vi "HFRR ADV v09.vi"() -> ()   [LabVIEW 2025] (continued)
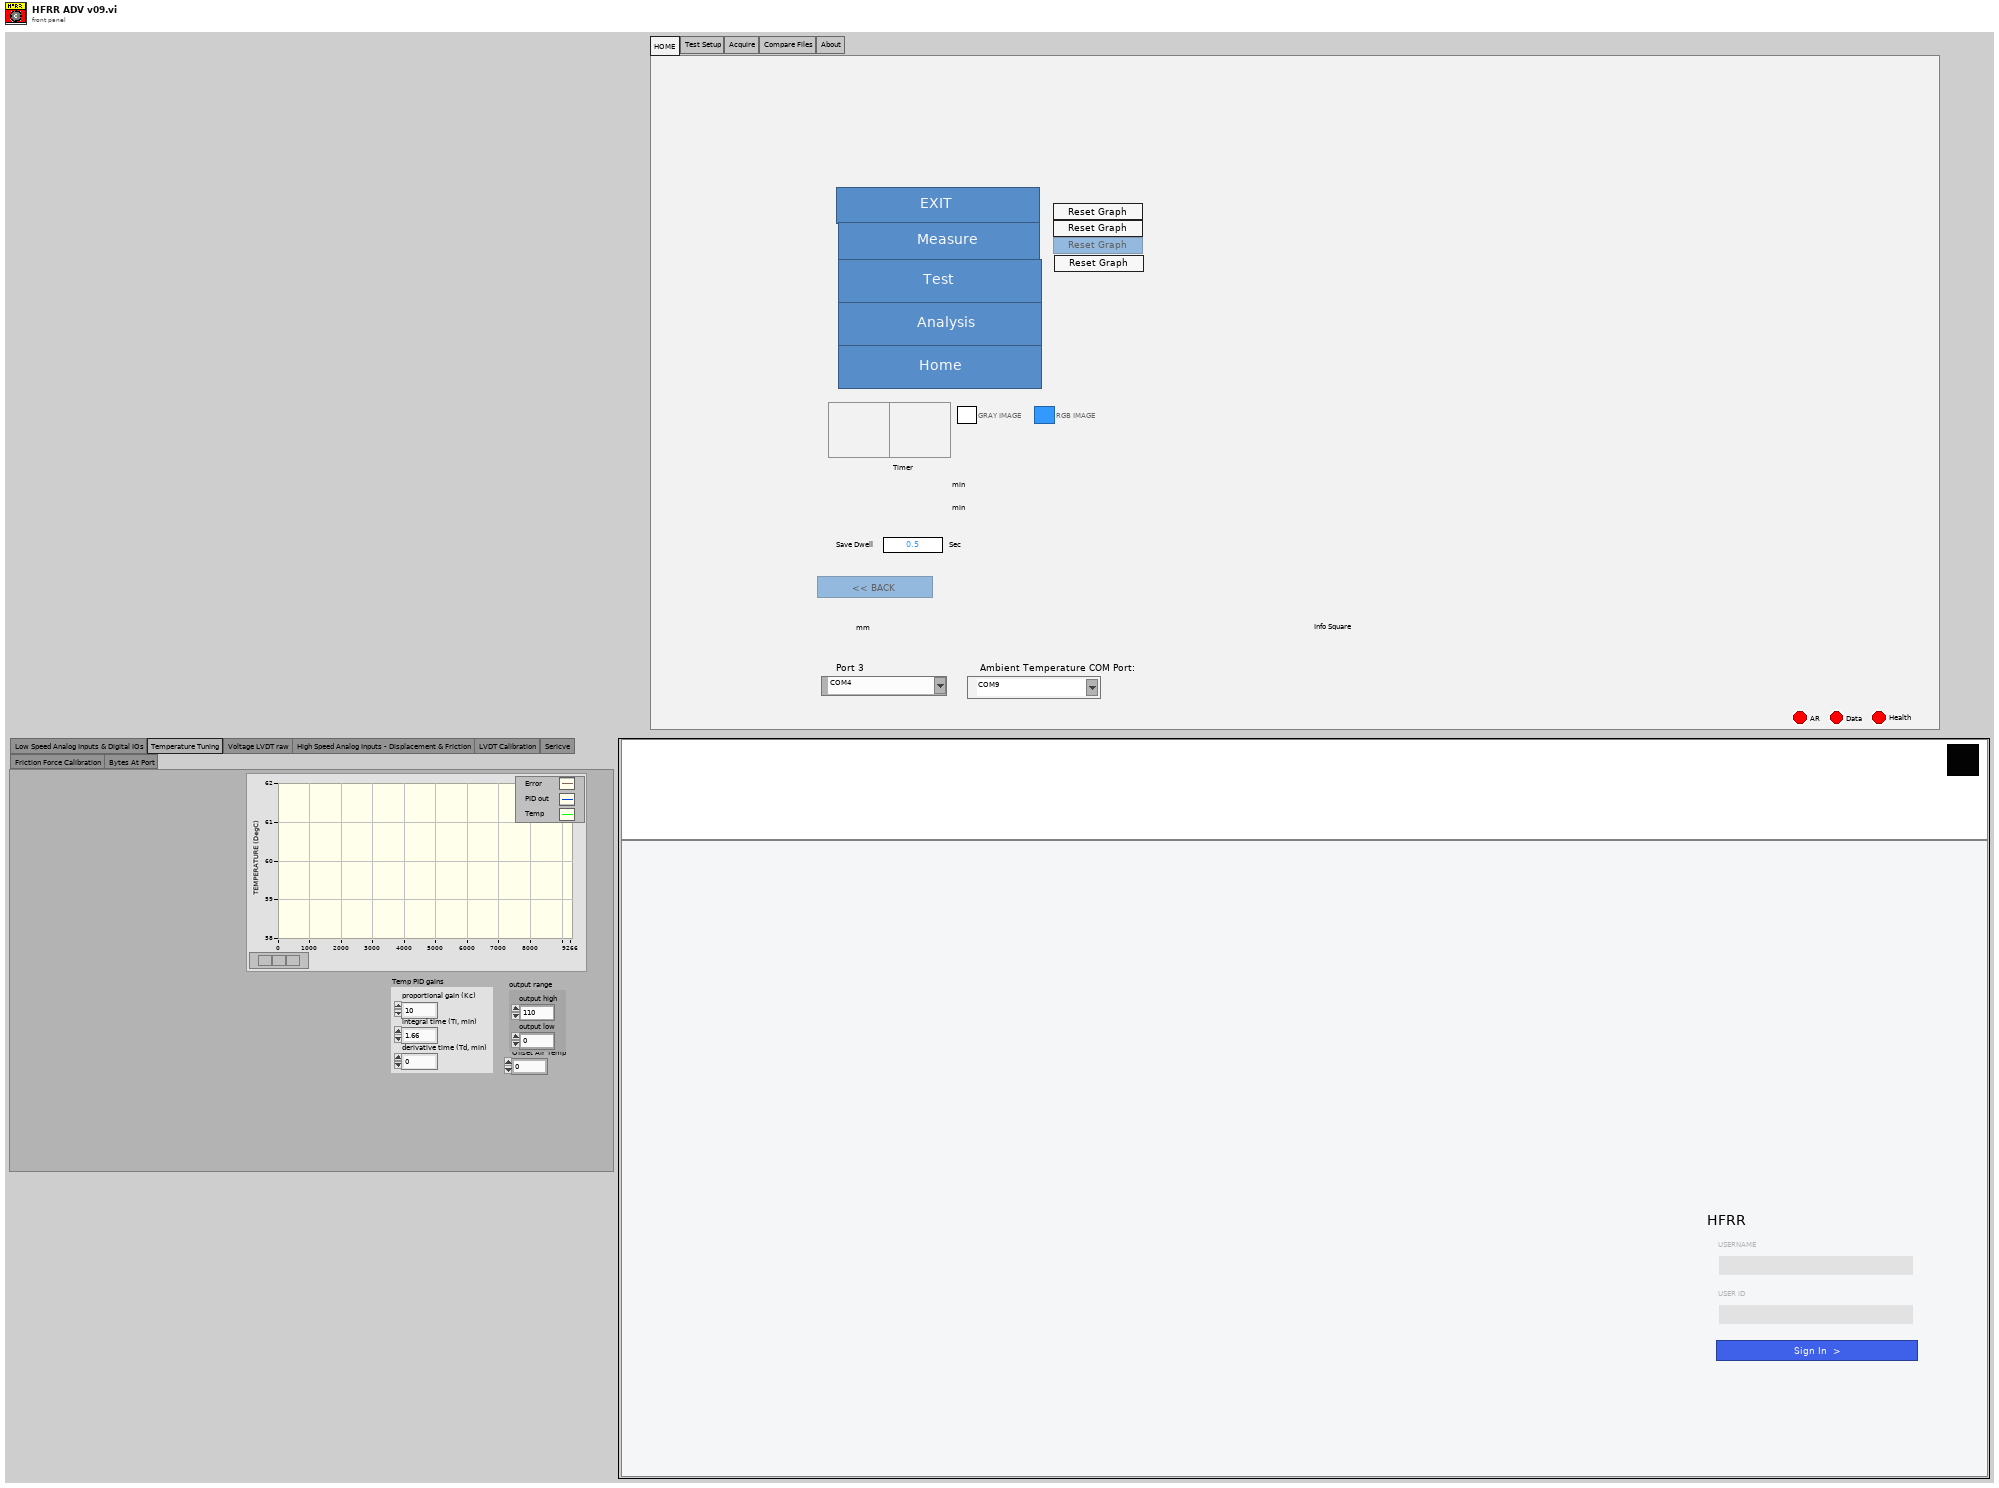
[diagram p1: front panel]
types:
  T1 = enum32{"Home", "Dashboard", "Imaging", "Report", "Analysis", "About", "Test Setup", "Advance"}
  T2 = enum32{"HOME", "Test Setup", "Acquire", "Adv Scar", "Adv Scar Report", "Compare Files", "About", "Advance", "Mooha"}
  T3 = enum16{"ASTM D6079", "ISO 12156", "CEC F-096-A-06", "Custom"}
  T4 = enum32{"Dashboard 1", "Dashboard 2", "Dashboard 3"}
  T5 = enum32{"COF", "Friction", "ECR", "Temperature", "Humidity", "Stroke"}
  T6 = enum32{"Coefficient Of Friction", "Air Temperature", "Humidity", "Stroke", "Sample Temperature", "Electrical Contact Resistance", "Frequency", "Air Temp vs Rh"}
  T7 = enum32{"Stroke Data", "Temperature Calibration", "Friction Force Raw Data"}
  T8 = cluster{"Proportional Gain (Kc)":dbl, "Integral Time (Ti, min)":dbl, "Derivative Time (Td, min)":dbl}
  T9 = enum32{"Temp Variables", "Camera", "WO 2465 (1)", "WO 2465 (2)", "WO 2465 (3)"}
  T10 = typedef "Auto Start enum.ctl" = enum16{"Init", "Humidity & Temperature On", "Reach point", "Maintain Stage", "Start Stage", "close", "Exit"}
  T11 = enum32{"Freqz control", "Low Speed Analog Inputs & Digital IOs", "Temperature Tuning", "Voltage LVDT raw", "High Speed Analog Inputs - Displacement & Friction", "LVDT Calibration", "Sericve", "Friction Force Calibration", "Bytes At Port", "Loadcell Board"}
  T12 = cluster{"proportional gain (Kc)":dbl, "integral time (Ti, min)":dbl, "derivative time (Td, min)":dbl}
  T13 = typedef "imagedata.ctl" = cluster{"image type":i32, "image depth":i32, "image":u8[], "mask":u8[], "colors":u32[], "Rectangle":cluster{"left":i16, "top":i16, "right":i16, "bottom":i16}}
  T14 = enum32{"HOME", "Test Setup", "Acquire", "Compare Files", "Print Report", "About", "Advance", "Mooha"}
  T15 = enum8{"Enabled", "Disabled", "Disabled and Grayed Out"}
  T16 = cluster{"Read Heave and Surge":string, "Bytes at Heave Port":dbl, "Heave and Surge COM Port:":refnum<visa-resource-name>, "Com Port 2":refnum<visa-resource-name>, "Residual Due":string, "Heave COM Status 2":bool, "Heave COM Status":bool, "Port 2":bool, "Sway PPR":dbl, "Surge PPR":dbl, "Heave PPR":dbl, "Sway Pitch":dbl, "Surge Pitch":dbl, "Heave Pitch":dbl, "Sway Pulses/mm":dbl, "Surge Pulses/mm":dbl, "Heave Pulses/mm":dbl, "inner loop":dbl, "Read Heave and Surge 2":string, "String 36":string, "Write S":bool, "WriteCC1":string[], "Heave COM Loop":i32, "LastCom":string, "EXIT":bool, "Error Heave":errorcluster}
  T17 = enum16{"Always On", "Always Off", "Off While Running"}
  T18 = typedef "POST ANALYSIS ENUM.ctl" = enum16{"OPEN EXE", "INIT", "OPEN FILE", "FIT", "DRAW REC", "DRAW LINE", "PAN", "ZOOM IN", "ZOOM OUT", "SET ZOOM", "CLEAR ROI", "GET MEASUREMENTS", "RESIZE MODE", "STREAM START", "STREAM STOP", "SHOW UI", "MINIMIZE UI", "HIDE UI", "CKISE APP", "CLOSE CONNECTION", "SAVE IMAGE", "SET ROI COLOR", "READ", "TCP CHECK", "CLOSE"}
  T19 = typedef "CAMERA LIVE FEED ENUM.ctl" = enum16{"OPEN EXE", "INIT", "READ", "CAMERA CONNECT", "CAMERA START", "CAMERA STOP", "CAMERA GRAY", "CAMERA RGB", "CAMERA MINIMIZE", "CAMERA CLOSE", "CAMERA MODE LIST", "CAMERA MODE SET", "CAMERA RESTORE", "CAMERA SAVE", "CLOSE"}
  T20 = cluster{"File Name":string, "Test Method":string, "Operator":string, "Fuel Description":string, "Date and time":string}
  T21 = enum32{"Home", "Dashboard", "Imaging", "Report", "Analysis", "About", "Test Setup"}
  T22 = enum32{"HOME", "Test Setup", "Acquire", "Compare Files", "About", "Advance", "Mooha"}
  T23 = enum16{"deny read/write", "deny write-only", "deny none"}
  T24 = typedef "NI_ReportGenerationCore.lvlib/HTML Report Image Alignment.ctl" = enum16{"(default)", "LEFT", "RIGHT", "TOP", "TEXTTOP", "MIDDLE", "ABSMIDDLE", "BASELINE", "BOTTOM", "ABSBOTTOM"}
  T25 = enum16{"open", "replace", "create", "open or create", "replace or create", "replace or create with confirmation"}
  T26 = enum16{"INIT", "READ", "MANUAL WRITE", "WRITE", "CLOSE", "ERROR INIT"}
  T27 = enum16{"open", "open or create", "create or replace", "create", "open (read only)"}
  T28 = cluster{"Mode":enum16{"RTU", "ASCII"}, "Slave Address":u8}
diagram:
  w1 = T15."Enabled" ("Disabled")
  w4 = FALSE ("Visible")
  w3 = FALSE ("Humidity Off Command")
  w23 = "" ("USER ID")
  # "[CH1]    - FF\n[CH2]   - TEMPERATURE\n[CH3]    - Humidity\n[CH4]    - AIR TEMP\n[CH5]\\- Visa Uno\n[CH6] \\- Visa Due\n[CH7]  \\- file path\n[CH8]   - Displacement Gain\n[CHA]   - Stroke Gain\n[CHB]   - Stroke PID Gain\n[CHC]   -Language Selection\n[CHD]   -Power +\n[CHE]   -Power_\n[CHF]   -Heater\n[CHG]   -Humidity Wet\n[CHH]   -Humidity Dry\n[CHI]   -Integral Time \n[CHIJ   -Air intercept\n[CHI]   -Temp Intercept"
  n1 = flat-sequence {
    tunnel: [w78] -> w14
    tunnel: w14 -> [w92]
    tunnel: [w91] -> w13
    tunnel: ["ao0"] -> w16
    tunnel: w13 -> [_]
    tunnel: w16 -> [w157]
    tunnel: [w157] -> w15
    tunnel: w15 -> [w210]
    tunnel: [w208] -> w27
    tunnel: [w210] -> w26
    tunnel: w27 -> [w261]
    tunnel: w26 -> [w217]
    tunnel: [w261] -> w12
    tunnel: [w223] -> w11
    tunnel: [w211] -> w10
    tunnel: [w268] -> _
    tunnel: [w267] -> _
    tunnel: [w269] -> w55
    tunnel: w12 -> [w269]
    tunnel: w11 -> [w267]
    tunnel: w10 -> [w268]
    frame #0 {
      n2 = control-ref of="This VI"() -> (w66:refnum<vi>)
      n3 = property class="VI"(reference=w66) -> (reference out=w57:refnum<vi>, error out=w61:errorcluster, "Panel"=w65:refnum<vi>)  [unwired: 1 in]
      n4 = property class="Pnl"(reference=w65, error in=w61) -> (reference out=w59:refnum<vi>, error out=w62:errorcluster, "Panes[]"=w64:refnum<vi>[])
      n5 = for {
        tunnel: w64 -> [w72] mode=indexing
        tunnel: T17."Always Off" ("Horizontal Scrollbar Visibility") -> [w71]
        tunnel: w62 -> [w68]
        tunnel: [w67] -> w60
        n6 = property class="Pane"(reference=w72, error in=w68, "HorizScrollbarVisibility"=w71) -> (reference out=w69:refnum<vi>, error out=w70:errorcluster)
        n7 = Close Reference(reference=w69, error in (no error)=w70) -> (error out=w67:errorcluster)
      }
      n8 = Close Reference(reference=w59, error in (no error)=w60) -> (error out=w58:errorcluster)
      n9 = Close Reference(reference=w57, error in (no error)=w58) -> (error out=→"error out 8":errorcluster)
    }
    frame #1 {
      n10 = call "CLOSE CONNECTION.vi"("error in (no error)"="error in (no error) 2") -> ("error out"=w76:errorcluster)  [unwired: 10 in]
      n11 = call <vilib>:"Clear Errors.vi"("error in (no error)"=w76) -> ("error out"=w75:errorcluster)  [unwired: 5 in, 1 out]
      n12 = disable-structure shown="Enabled" {
        disable-tunnel: w75 -> [w82 _]
        disable-tunnel: [w81 _] -> w78
        frame Enabled {
          n13 = call <userlib>:"Fit VI window to Largest Dec.vi"("error in (no error)"=w82, "border spacing (2 px)"=1) -> ("error out"=w85:errorcluster, "dup VI Ref"=w89:refnum<vi>)  [unwired: 4 in]
          n14 = invoke on="Invoke Node" class="VI" method="FP.Run-Time Position.Maximized"(reference=w89, error in=w85) -> (error out=w86:errorcluster)  [unwired: 2 in, 3 out]
          n15 = call <vilib>:"Clear Errors.vi"("error in (no error)"=w86) -> ("error out"=w88:errorcluster)  [unwired: 5 in, 1 out]
          n16 = control-ref of="This VI"() -> (w80:refnum<vi>)
          n17 = invoke on="Invoke Node" class="VI" method="Default Vals.Reinit All"(reference=w80, error in=w88) -> (reference out=w84:refnum<vi>, error out=w83:errorcluster)  [unwired: 1 in, 1 out]
          n18 = Close Reference(reference=w84, error in (no error)=w83) -> (error out=w81:errorcluster)
        }
        frame Disabled {
        }
      }
      n19 = local write "sign in temp"(FALSE ("sign in temp")) -> ()
      n20 = property on="Sign In" class="Bool (strict)"("DisabledEnum"=T15."Disabled" ("Disabled")) -> ()  [unwired: 2 in, 2 out]
      n21 = property on="Auto Scar Check" class="Clust (strict)"("Visible"=TRUE) -> ()  [unwired: 2 in, 2 out]
    }
    frame #2 {
      n22 = call "dialog box.vi"("Status"="Before starting the test, verify that the microscope cable is connected.", "error in"=w92) -> ("error out"=w91:errorcluster)  [unwired: 8 in]
    }
    frame #3 {
      w99 = FALSE ("Upld AR 2")
      # "kkkkk"
      # "C:\\Windows\\wndcm_pw_stdED hfrr.txt"
      # "C:\\LAB-IQ NXT"
      # "C:\\LAB-IQ NXT\\wndcm_pw_stdED hfrr.txt"
      # "password file"
      n23 = Current VI's Path() -> (path=w112:path)
      n24 = Strip Path(path=w112) -> (stripped path=w105:path)  [unwired: 1 out]
      n25 = Path To String(path=w105) -> (string=w107:string)
      n26 = local write "conststatus"(0.0 ("rpm value : 2")) -> ()
      n27 = local write "Upld AR 2"(TRUE ("Upld AR 2")) -> ()
      n28 = local write "Lan flag"(0.0 ("Lan flag")) -> ()
      n29 = local write "COUNT"(0 ("COUNT")) -> ()
      n30 = local write "FLAG 2"(0.0 ("FLAG 2")) -> ()
      n31 = local write "Com flag"(u32 0 ("Com flag")) -> ()
      n32 = local write "Re-Initialise"(TRUE ("Re-Initialise")) -> ()
      n33 = local write "refresh flag"(FALSE ("refresh flag")) -> ()
      n34 = local write "Json St Flg"(w99) -> ()
      n35 = Search/Split String(string=w107, search string/char (-)=".exe") -> (match + rest of string=w109:string)  [unwired: 1 in, 2 out]
      n36 = Match True/False String(2:".vi" ("false string"), 3:".exe" ("true string"), 4:w109) -> (0:w106:bool)  [unwired: 1 out]
      n37 = local write "Json End Flg"(w99) -> ()
      n38 = case shown="True" w106 {
        tunnel: w105 -> [w128 w130]
        tunnel: [w128 w129] -> w103
        frame False {
        }
        frame True {
          n39 = Strip Path(path=w130) -> (stripped path=w129:path)  [unwired: 1 out]
        }
      }
      n40 = Path To String(path=w103) -> (string=→"Gain path":string)
      n41 = local write "Main Tab Display"(T4."Dashboard 1" ("Main Tab Display")) -> ()
      n42 = local write "main tab sub"(enum32{"Page 1", "Page 2"}."Page 1" ("main tab sub")) -> ()
      n43 = local write "Main Tab"(T2."HOME" ("Main Tab")) -> ()
      n44 = local write "EVENT LOG"("") -> ()
      n45 = List Folder(path=path "C:/LAB-IQ" ("directory path"), pattern="*.txt") -> (filenames=w118:string[])  [unwired: 2 in, 3 out]
      n46 = Search 1D Array(1D array=w118, element="wndcm_pw_stdED hfrr.txt") -> (index of element=w121:i32)  [unwired: 1 in]
      n47 = Equal?(x=w121, y=-1) -> (x = y?=w116:bool)
      n48 = case shown="True" w116 {
        frame False {
        }
        frame True {
          n49 = String To Byte Array(string="123\n") -> (unsigned byte array=w135:u8[])
          n50 = Array Size(array=w135) -> (size(s)=w134:i32)
          n51 = for {
            N: w134 -> [_]
            tunnel: w135 -> [w148]
            tunnel: [w145] -> w137 mode=indexing
            tunnel: w134 -> [w140]
            i -> [w138]
            n52 = Decrement(x=w140) -> (x-1=w141:i32)
            n53 = Equal?(x=w138, y=w141) -> (x = y?=w142:bool)
            n54 = Index Array(array=w148, index=w138) -> (element=w147:u8)
            n55 = Number To Decimal String(number=w147) -> (decimal integer string=w146:string)  [unwired: 1 in]
            n56 = Select(t="", s=w142, f="\r") -> (s? t:f=w139:string)
            n57 = Concatenate Strings(w146, w139) -> (w145:string)
          }
          n58 = local read "file path"() -> (w131:path)
          n59 = Concatenate Strings(w137) -> (w133:string)
          n60 = call <vilib>:"Write Characters To File.vi"("append to file? (new file:F)"=FALSE, "character string"=w133, "file path (dialog if empty)"=w131) -> ()  [unwired: 2 in, 1 out]
        }
      }
      n61 = local write "clk"(0.0 ("clk")) -> ()
      n62 = local write "Flag"(0.0 ("Flag")) -> ()
      "file path" <- path "C:/LAB-IQ/wndcm_pw_stdED hfrr.txt" ("file path")
      "FF buffer" <- dbl[] [] ("FF buffer")
    }
    frame #4 {
      # "C:\\WinDucom\\calibrate WO 2391.dcf"
      n63 = String To Path(string="C:\\LAB-IQ\\calibrate WO 2465.dcf") -> (path=w156:path)
      n64 = Open/Create/Replace File "Open File"(file path (use dialog)=w156) -> (refnum out=w155:refnum<file>)  [unwired: 5 in, 2 out]
      n65 = for {
        N: 24 -> [_]
        tunnel: w155 -> [w176]
        i -> [w170]
        (unwired) TRUE ("line mode (F)")
        n66 = Read from Text File "Read File"(file (use dialog)=w176) -> (text=w175:string)  [unwired: 3 in, 3 out]
        n67 = Match Pattern(string=w175, regular expression="]") -> (after substring=w173:string)  [unwired: 1 in, 3 out]
        n68 = String Subset(string=w175, offset (0)=5, length (rest)=10 ("length (rest)")) -> (substring=w168:string)
        n69 = Fract/Exp String To Number(string=w168) -> (number=w169:dbl)  [unwired: 3 in, 1 out]
        n70 = Match Pattern(string=w173, regular expression="-") -> (before substring=w171:string)  [unwired: 1 in, 3 out]
        n71 = case shown="7" w170 {
          tunnel: w169 -> [w179 w180 w181 w182 _ _ _ w187 w188 w189 w192 w193 w194 w195 w196 w197 w198 w201 w202 _ _ w205 _ _ _]
          tunnel: w171 -> [_ _ _ _ w183 w184 w185 _ _ _ _ _ _ _ _ _ _ _ _ w203 w204 _ w206 w207 _]
          frame 0 {
            n72 = local write "FRIC. FORCE :"(w179) -> ()
          }
          frame 1 {
            n73 = local write "TEMPERATURE :"(w180) -> ()
          }
          frame 2 {
            n74 = local write "HUMIDITY:"(w181) -> ()
          }
          frame 3 {
            n75 = local write "AIR TEMPERATURE :"(w182) -> ()
          }
          frame 4 {
            n76 = local write "Com Port 1"(w183) -> ()
          }
          frame 5 {
            n77 = local write "Com Port 2"(w184) -> ()
            n78 = local write "visa due"(w184) -> ()
          }
          frame 6 {
            n79 = String To Path(string=w185) -> (path=w186:path)
            n80 = local write "File Path"(w186) -> ()
          }
          frame 7 {
            n81 = local write "DISPLACEMENT :"(w187) -> ()
          }
          frame 8 {
            n82 = local write "STROKE GAIN :"(w188) -> ()
          }
          frame 9 {
            n83 = local read "Stroke PID Gains"() -> (w191:T8)
            n84 = Bundle By Name(cluster=w191, "Proportional Gain (Kc)"=w189) -> (w190:T8)
            n85 = local write "Stroke PID Gains"(w190) -> ()
          }
          frame 10 {
            n86 = local write "Language Selection"(w192) -> ()
          }
          frame 11 {
            n87 = local write "CH-POWER +"(w193) -> ()
          }
          frame 12 {
            n88 = local write "CH-POWER -"(w194) -> ()
          }
          frame 13 {
            n89 = local write "CH-HEATER"(w195) -> ()
          }
          frame 14 {
            n90 = local write "CH-HUMIDITY WET"(w196) -> ()
          }
          frame 15 {
            n91 = local write "CH-HUMIDITY DRY"(w197) -> ()
          }
          frame 16 {
            n92 = local read "Stroke PID Gains"() -> (w200:T8)
            n93 = Bundle By Name(cluster=w200, "Integral Time (Ti, min)"=w198) -> (w199:T8)
            n94 = local write "Stroke PID Gains"(w199) -> ()
          }
          frame 17 {
            n95 = local write "AIR TEMP INTERCEPT:"(w201) -> ()
          }
          frame 18 {
            n96 = local write "TEMP INTERCEPT:"(w202) -> ()
          }
          frame 19 {
            n97 = local write "S.NO"(w203) -> ()
          }
          frame 20 {
            n98 = local write "Com Port 3"(w204) -> ()
          }
          frame 21 {
            n99 = local write "LvdtOff"(w205) -> ()
          }
          frame 22 {
            n100 = local write "Humidity :"(w206) -> ()
          }
          frame 23 {
            n101 = local write "Camera Port :"(w207) -> ()
          }
          frame 24, Default {
          }
        }
      }
      n102 = String To Path(string="C:\\LAB-IQ\\Image Calibrate v01.dcf") -> (path=w152:path)
      n103 = Open/Create/Replace File ("Open File")(file path (use dialog)=w152) -> (refnum out=w151:refnum<file>)  [unwired: 5 in, 2 out]
      n104 = for {
        N: 4 -> [_]
        tunnel: w151 -> [w163]
        i -> [w159]
        n105 = Read from Text File ("Read File")(file (use dialog)=w163) -> (text=w164:string)  [unwired: 3 in, 3 out]
        n106 = String Subset(string=w164, offset (0)=6, length (rest)=10 ("length (rest)")) -> (substring=w160:string)
        n107 = Fract/Exp String To Number(string=w160) -> (number=w158:dbl)  [unwired: 3 in, 1 out]
        n108 = case shown="3" w159 {
          tunnel: w158 -> [w165 w166 _ w167 _]
          frame 0 {
            n109 = local write "5x Gain"(w165) -> ()
          }
          frame 1 {
            n110 = local write "10x Gain"(w166) -> ()
          }
          frame 2 {
          }
          frame 3 {
            n111 = local write "100x gain"(w167) -> ()
          }
          frame 4, Default {
          }
        }
      }
    }
    frame #5 {
      n112 = Wait (ms)(milliseconds to wait=u32 1000) -> (millisecond timer value=w208:u32)
    }
    frame #6 {
      w226 = u32 2000 ("milliseconds to wait")
      w253 = u32 2000 ("milliseconds to wait")
      n113 = local read "Re-Initialise"() -> (w260:bool)
      n114 = case shown="True" w260 {
        frame False {
        }
        frame True {
          n115 = local write "Re-Initialise"(FALSE ("Re-Initialise")) -> ()
        }
      }
      n116 = call "CAMERA LIVE FEED FGV.vi"("Enum - Menu"=CAMERA_LIVE_FEED_ENUM."OPEN EXE", "error in (no error)"=w217) -> ("error out"=w259:errorcluster)  [unwired: 8 in, 1 out]
      n117 = call "Stall Data Flow.vim"("value in"=w259, "milliseconds to wait"=w253) -> ("value out"=w257:errorcluster)  [unwired: 1 out]
      n118 = call "CAMERA LIVE FEED FGV.vi"("Enum - Menu"=CAMERA_LIVE_FEED_ENUM."INIT", "error in (no error)"=w257) -> ("error out"=w255:errorcluster)  [unwired: 8 in, 1 out]
      n119 = call "IMAGE ANALYSIS.vi"("Enum"=POST_ANALYSIS_ENUM."OPEN EXE", "error in"=w217) -> ("error out"=w214:errorcluster)  [unwired: 8 in, 1 out]
      n120 = case shown="Error .." w255 {
        selector: w255 -> [w262 _]
        tunnel: [w262 _] -> w254
        frame No Error {
        }
        frame Error {
          n121 = One Button Dialog(message="Camera initialization error.\nPlease Restart the software") -> ()  [unwired: 1 in, 1 out]
        }
      }
      n122 = call "Stall Data Flow.vim"("value in"=w214, "milliseconds to wait"=u32 8000) -> ("value out"=w213:errorcluster)  [unwired: 1 out]
      n123 = property on="Camera Port :" class="CmbBox"() -> ("Strings[]"=w251:string[], "Value"=w252:string)  [unwired: 2 in, 2 out]
      n124 = call "IMAGE ANALYSIS.vi"("Enum"=POST_ANALYSIS_ENUM."INIT", "error in"=w213) -> ("error out"=w211:errorcluster)  [unwired: 8 in, 1 out]
      n125 = Search 1D Array(1D array=w251, element=w252) -> (index of element=w250:i32)  [unwired: 1 in]
      n126 = Type Cast(type=30, x=w250) -> (*(type *) &x=w248:i32)
      n127 = call "Stall Data Flow.vim"("value in"=w254, "milliseconds to wait"=w253) -> ("value out"=w230:errorcluster)  [unwired: 1 out]
      n128 = Add(x=w248, y=48) -> (x+y=w229:i32)
      n129 = call "CAMERA LIVE FEED FGV.vi"("Enum - Menu"=CAMERA_LIVE_FEED_ENUM."CAMERA CONNECT", "error in (no error)"=w230, "CAMERA PORT"=w229) -> ("error out"=w239:errorcluster)  [unwired: 7 in, 1 out]
      n130 = call "Stall Data Flow.vim"("value in"=w239, "milliseconds to wait"=u32 5000) -> ("value out"=w240:errorcluster)  [unwired: 1 out]
      n131 = call "CAMERA LIVE FEED FGV.vi"("Enum - Menu"=CAMERA_LIVE_FEED_ENUM."CAMERA MODE LIST", "error in (no error)"=w240) -> ("error out"=w242:errorcluster)  [unwired: 8 in, 1 out]
      n132 = call "Stall Data Flow.vim"("value in"=w242, "milliseconds to wait"=w226) -> ("value out"=w241:errorcluster)  [unwired: 1 out]
      n133 = Type Cast(type=30, x=0) -> (*(type *) &x=w222:i32)
      n134 = Add(x=w222, y=48) -> (x+y=w220:i32)
      n135 = call "CAMERA LIVE FEED FGV.vi"("Enum - Menu"=CAMERA_LIVE_FEED_ENUM."READ", "error in (no error)"=w241) -> ("error out"=w228:errorcluster, "data out"=→"Camera List":string)  [unwired: 8 in]
      n136 = call "Stall Data Flow.vim"("value in"=w228, "milliseconds to wait"=w226) -> ("value out"=w227:errorcluster)  [unwired: 1 out]
      n137 = call "CAMERA LIVE FEED FGV.vi"("Enum - Menu"=CAMERA_LIVE_FEED_ENUM."CAMERA MODE SET", "error in (no error)"=w227, "CAMERA MODE"=w220) -> ("error out"=w224:errorcluster)  [unwired: 7 in, 1 out]
      n138 = call "Stall Data Flow.vim"("value in"=w224, "milliseconds to wait"=u32 2000) -> ("value out"=w244:errorcluster)  [unwired: 1 out]
      n139 = call "CAMERA LIVE FEED FGV.vi"("Enum - Menu"=CAMERA_LIVE_FEED_ENUM."CAMERA START", "error in (no error)"=w244) -> ("error out"=w245:errorcluster)  [unwired: 8 in, 1 out]
      n140 = call "Stall Data Flow.vim"("value in"=w245, "milliseconds to wait"=u32 1000) -> ("value out"=w246:errorcluster)  [unwired: 1 out]
      n141 = call "CAMERA LIVE FEED FGV.vi"("Enum - Menu"=CAMERA_LIVE_FEED_ENUM."CAMERA MINIMIZE", "error in (no error)"=w246) -> ("error out"=w223:errorcluster)  [unwired: 8 in, 1 out]
    }
    frame #7 {
      n142 = case shown="No Error" w267 {
        frame No Error {
          n143 = property on="Auto Scar Check" class="Clust (strict)"("Visible"=FALSE) -> ()  [unwired: 2 in, 2 out]
        }
        frame Error {
        }
      }
      n144 = local write "sign in temp"(TRUE ("sign in temp")) -> ()
      n145 = property on="Sign In" class="Bool (strict)"("DisabledEnum"=T15."Enabled" ("Disabled")) -> ()  [unwired: 2 in, 2 out]
    }
  }
  n146 = property on="Auto Start Test" class="Bool (strict)"("Visible"=TRUE) -> ()  [unwired: 2 in, 2 out]
  n147 = property on="FRICVALZ 2" class="Bool (strict)"("DisabledEnum"=w1) -> ()  [unwired: 2 in, 2 out]
  n148 = property on="FRICVALZ 4" class="Bool (strict)"("DisabledEnum"=w1) -> ()  [unwired: 2 in, 2 out]
  n149 = property on="FRICVALZ 3" class="Bool (strict)"("DisabledEnum"=w1) -> ()  [unwired: 2 in, 2 out]
  n150 = property on="About" class="Clust (strict)"("Visible"=FALSE) -> ()  [unwired: 2 in, 2 out]
  n151 = local write "Temperature Off Command"(w3) -> ()
  n152 = local write "Main Dashboard Buttons"(T1."Home" ("Main Dashboard Buttons")) -> ()
  n153 = local write "Humidity Off Command"(w3) -> ()
  n154 = local write "CAMERA ROI MIN TEMP"(w3) -> ()
  n155 = local write "TEST FILE NAM,E SAVED"(w3) -> ()
  n156 = local write "LIVE FEED MIN TEMP"(w3) -> ()
  n157 = while {
    shift-right: [w272] -> _
    shift-left: "Enum - Selector" -> [w273]
    stop <- w274 stop-if-true
    # "Auto Start Logic Loop"
    n158 = case shown="\"Maintain Stage\"" w273 {
      tunnel: [w277 w283 w294 w326 w357 Auto_Start_enum."Exit" ("Enum - Selector") Auto_Start_enum."Init" ("Enum - Selector")] -> w272
      frame "Init", Default {
        n159 = local read "Auto Start Test"() -> (w276:bool)
        n160 = Select(t=Auto_Start_enum."Humidity & Temperature On" ("Enum - Selector"), s=w276, f=Auto_Start_enum."Init") -> (s? t:f=w277:T10)
      }
      frame "Humidity & Temperature On" {
        n161 = flat-sequence {
          tunnel: [Auto_Start_enum."Reach point" ("Enum - Selector")] -> w280
          frame #0 {
            w284 = T15."Disabled and Grayed Out" ("Disabled")
            w285 = TRUE ("Heater Button")
            n162 = property on="Humidity" class="Bool (strict)"("DisabledEnum"=w284) -> ()  [unwired: 2 in, 2 out]
            n163 = property on="Heater Button" class="Bool (strict)"("DisabledEnum"=w284) -> ()  [unwired: 2 in, 2 out]
            n164 = local write "Heater Button"(w285) -> ()
            n165 = local write "Humidity"(w285) -> ()
          }
          frame #1 {
            n166 = Wait (ms)(milliseconds to wait=u32 1000) -> ()  [unwired: 1 out]
          }
          frame #2 {
            w287 = TRUE ("Reach point temp")
            n167 = local write "Reach point Humidity"(w287) -> ()
            n168 = local write "Reach point temp"(w287) -> ()
          }
        }
        n169 = local read "Auto Start Test"() -> (w282:bool)
        n170 = Not(x=w282) -> (.not. x?=w281:bool)
        n171 = Select(t=Auto_Start_enum."close", s=w281, f=w280) -> (s? t:f=w283:T10)
      }
      frame "Reach point" {
        w295 = TRUE ("PAUSE")
        w303 = 1.0 ("y")
        w306 = 1.0 ("y")
        n172 = local read "Set Temperature:"() -> (w307:dbl)
        n173 = local read "Set Humidity:"() -> (w302:dbl)
        n174 = local read "Humidity ( %RH )"() -> (w308:dbl)
        n175 = Add(x=w307, y=w306) -> (x+y=w305:dbl)
        n176 = Subtract(x=w307, y=w306) -> (x-y=w304:dbl)
        n177 = Add(x=w302, y=w303) -> (x+y=w301:dbl)
        n178 = Subtract(x=w302, y=w303) -> (x-y=w300:dbl)
        n179 = local read "TEMP"() -> (w309:dbl)
        n180 = In Range and Coerce(upper limit=w301, x=w308, lower limit=w300) -> (In Range?=w289:bool)  [unwired: 1 out]
        n181 = In Range and Coerce(upper limit=w305, x=w309, lower limit=w304) -> (In Range?=w290:bool)  [unwired: 1 out]
        n182 = case shown="True" w289 {
          frame False {
          }
          frame True {
            n183 = case shown="True" "Reach point Humidity" {
              selector: "Reach point Humidity" -> [_ w315]
              frame False {
              }
              frame True {
                n184 = local read "EVENT LOG"() -> (w312:string)
                n185 = Not(x=w315) -> (.not. x?=w314:bool)
                n186 = local write "Reach point Humidity"(w314) -> ()
                n187 = call "Event Log.vi"("Content"="Target Humidity reached", "EVENT LOG"=w312) -> ("EVENT LOG"=w313:string)  [unwired: 8 in, 1 out]
                n188 = local write "EVENT LOG"(w313) -> ()
              }
            }
          }
        }
        n189 = case shown="True" w290 {
          frame False {
          }
          frame True {
            n190 = case shown="True" "Reach point temp" {
              selector: "Reach point temp" -> [_ w321]
              frame False {
              }
              frame True {
                n191 = local read "EVENT LOG"() -> (w318:string)
                n192 = Not(x=w321) -> (.not. x?=w320:bool)
                n193 = local write "Reach point temp"(w320) -> ()
                n194 = call "Event Log.vi"("Content"="Target Temperature reached", "EVENT LOG"=w318) -> ("EVENT LOG"=w319:string)  [unwired: 8 in, 1 out]
                n195 = local write "EVENT LOG"(w319) -> ()
              }
            }
          }
        }
        n196 = local read "Auto Start Test"() -> (w293:bool)
        n197 = And(x=w290, y=w289) -> (x .and. y?=w299:bool)
        n198 = Select(t=Auto_Start_enum."Maintain Stage" ("Enum - Selector"), s=w299, f=Auto_Start_enum."Reach point" ("Enum - Selector")) -> (s? t:f=w296:T10)
        n199 = Not(x=w293) -> (.not. x?=w292:bool)
        n200 = Select(t=Auto_Start_enum."close", s=w292, f=w296) -> (s? t:f=w294:T10)
        n201 = call "ELAPSED TIMER VI.vi"("RESET"=w295, "PAUSE"=w295) -> ()  [unwired: 7 in, 3 out]
      }
      frame "Maintain Stage" {
        w335 = 1.0 ("y")
        w334 = 1.0 ("y")
        # "Humidity and  temperatures Set Point  have been reached"
        n202 = local read "Set Temperature:"() -> (w341:dbl)
        n203 = local read "Set Humidity:"() -> (w338:dbl)
        n204 = local read "Humidity ( %RH )"() -> (w342:dbl)
        n205 = Add(x=w341, y=w334) -> (x+y=w340:dbl)
        n206 = Subtract(x=w341, y=w334) -> (x-y=w339:dbl)
        n207 = local read "TEMP"() -> (w343:dbl)
        n208 = Add(x=w338, y=w335) -> (x+y=w337:dbl)
        n209 = Subtract(x=w338, y=w335) -> (x-y=w336:dbl)
        n210 = In Range and Coerce(upper limit=w340, x=w343, lower limit=w339) -> (In Range?=w333:bool)  [unwired: 1 out]
        n211 = In Range and Coerce(upper limit=w337, x=w342, lower limit=w336) -> (In Range?=w332:bool)  [unwired: 1 out]
        n212 = And(x=w333, y=w332) -> (x .and. y?=w331:bool)
        n213 = Not(x=w331) -> (.not. x?=w330:bool)
        n214 = call "ELAPSED TIMER VI.vi"("TARGET"=60.0, "RESET"=w330, "PAUSE"=FALSE) -> ("ELAPSED INDICATION"=w327:bool)  [unwired: 6 in, 2 out]
        n215 = case shown="True" w327 {
          tunnel: w327 -> [_ w346]
          tunnel: [Auto_Start_enum."Maintain Stage" ("Enum - Selector") w345] -> w325
          frame False {
          }
          frame True {
            n216 = stacked-sequence {
              tunnel: w346 -> [_ _ _ _ _]
              tunnel: [_ _ _ _ Auto_Start_enum."Start Stage" ("Enum - Selector")] -> w345
              frame #0 {
                n217 = local read "EVENT LOG"() -> (w348:string)
                n218 = call "Event Log.vi"("Content"="Humidity and temperature set point has stabilized.", "EVENT LOG"=w348) -> ("EVENT LOG"=w349:string)  [unwired: 8 in, 1 out]
                n219 = local write "EVENT LOG"(w349) -> ()
              }
              frame #1 {
                n220 = Wait (ms)(milliseconds to wait=u32 100) -> ()  [unwired: 1 out]
              }
              frame #2 {
                n221 = local read "EVENT LOG"() -> (w352:string)
                n222 = call "Event Log.vi"("Content"="Auto Test Started", "EVENT LOG"=w352) -> ("EVENT LOG"=w353:string)  [unwired: 8 in, 1 out]
                n223 = local write "EVENT LOG"(w353) -> ()
              }
              frame #3 {
                w354 = TRUE ("RUN")
                n224 = local write "RUN"(w354) -> ()
                "Auto Start Temp" <- w354
              }
              frame #4 {
              }
            }
          }
        }
        n225 = local read "Auto Start Test"() -> (w324:bool)
        n226 = Not(x=w324) -> (.not. x?=w323:bool)
        n227 = Select(t=Auto_Start_enum."close", s=w323, f=w325) -> (s? t:f=w326:T10)
      }
      frame "Start Stage" {
        w356 = TRUE ("PAUSE")
        n228 = local read "Auto Start Test"() -> (w361:bool)
        n229 = Not(x=w361) -> (.not. x?=w360:bool)
        n230 = Select(t=Auto_Start_enum."close" ("Enum - Selector"), s=w360, f=Auto_Start_enum."Start Stage" ("Enum - Selector")) -> (s? t:f=w357:T10)
        n231 = call "ELAPSED TIMER VI.vi"("RESET"=w356, "PAUSE"=w356) -> ()  [unwired: 7 in, 3 out]
      }
      frame "close" {
        w362 = FALSE ("Heater Button")
        n232 = local write "RUN"(w362) -> ()
        n233 = local write "Heater Button"(w362) -> ()
        n234 = local write "Humidity"(w362) -> ()
        n235 = local write "Auto Start Test"(w362) -> ()
      }
      frame "Exit" {
      }
    }
    n236 = Wait (ms)(milliseconds to wait=u32 100) -> ()  [unwired: 1 out]
    n237 = local read "Quit"() -> (w274:bool)
  }
  n238 = while {
    stop <- w365 stop-if-true
    n239 = event shown="[3] \"Auto Start Test\": Value Change" {
      selector: _ -> [_ _ _ _ _ _ _ _ _ _ _]
      dyn-events: _ -> [_ _ _ _ _ _ _ _ _ _ _]
      timeout: 100 -> [_ _ _ _ _ _ _ _ _ _ _]
      tunnel: [FALSE FALSE _ FALSE _ _ _ _ _ _ TRUE] -> w365
      event Timeout {
        n240 = event-data() -> ()  [unwired: 1 in, 3 out]
        n241 = Get Date/Time In Seconds() -> (seconds since 1Jan1904=w376:timestamp)
        n242 = Format Into String(format string="%<%I:%M:%S:%p %d:%B:%Y>T", w376) -> (resulting string=→"Time Stamp":string)  [unwired: 2 in, 1 out]
        n243 = local read "FILE"() -> (w373:string)
        n244 = local read "Service Password enable"() -> (w368:bool)
        n245 = call <vilib>:"Trim Whitespace.vi"("string"=w373) -> ("trimmed string"=w372:string)  [unwired: 1 in]
        n246 = String Length(string=w372) -> (length=w371:i32)
        n247 = Greater?(x=w371, y=1) -> (0:w369:bool)
        n248 = case shown="False" w369 {
          tunnel: w368 -> [w378 _]
          frame False {
            n249 = case shown="True" w378 {
              frame True {
                w379 = "Test Start In Service Mode" ("Tip Strip")
                w380 = T15."Enabled" ("Disabled")
                n250 = property on="Auto Start Test" class="Bool (strict)"("DisabledEnum"=w380, "TipStrip"=w379) -> ()  [unwired: 2 in, 2 out]
                n251 = property on="RUN" class="Bool (strict)"("DisabledEnum"=w380, "TipStrip"=w379) -> ()  [unwired: 2 in, 2 out]
              }
              frame False {
                w381 = "Enter File Name to Start Test" ("Tip Strip")
                w382 = T15."Disabled and Grayed Out" ("Disabled")
                n252 = property on="Auto Start Test" class="Bool (strict)"("DisabledEnum"=w382, "TipStrip"=w381) -> ()  [unwired: 2 in, 2 out]
                n253 = property on="RUN" class="Bool (strict)"("DisabledEnum"=w382, "TipStrip"=w381) -> ()  [unwired: 2 in, 2 out]
              }
            }
          }
          frame True {
            w383 = "" ("Tip Strip")
            w384 = T15."Enabled" ("Disabled")
            n254 = property on="Auto Start Test" class="Bool (strict)"("DisabledEnum"=w384, "TipStrip"=w383) -> ()  [unwired: 2 in, 2 out]
            n255 = property on="RUN" class="Bool (strict)"("DisabledEnum"=w384, "TipStrip"=w383) -> ()  [unwired: 2 in, 2 out]
          }
        }
      }
      event "RUN": Value Change {
        n256 = event-data() -> ()  [unwired: 1 in, 6 out]
        n257 = local read "RUN"() -> (w386:bool)
        n258 = case shown="True" w386 {
          frame False {
            w387 = T15."Enabled" ("Disabled")
            w391 = "" ("FILE")
            n259 = local write "FILE"(w391) -> ()
            n260 = local write "Batch Ref Num :"(w391) -> ()
            n261 = local write "Fuel Discription :"(w391) -> ()
            n262 = local write "Main Tab"(T2."Adv Scar" ("Main Tab")) -> ()
            n263 = local write "Remarks :"(w391) -> ()
            n264 = local write "Main Dashboard Buttons"(T1."Imaging" ("Main Dashboard Buttons")) -> ()
            n265 = local write "TEST FILE NAM,E SAVED"(FALSE ("TEST FILE NAM,E SAVED")) -> ()
            n266 = property on="Stroke ( mm )" class="WFChart (strict)"("History Data"=cluster{"y":dbl, dbl, "y":dbl}[] []) -> ()  [unwired: 2 in, 2 out]
            n267 = property on="Auto Start Test" class="Bool (strict)"("Visible"=TRUE) -> ()  [unwired: 2 in, 2 out]
            n268 = property on="FRICVALZ 2" class="Bool (strict)"("DisabledEnum"=w387) -> ()  [unwired: 2 in, 2 out]
            n269 = property on="FRICVALZ 4" class="Bool (strict)"("DisabledEnum"=w387) -> ()  [unwired: 2 in, 2 out]
            n270 = property on="FRICVALZ 3" class="Bool (strict)"("DisabledEnum"=w387) -> ()  [unwired: 2 in, 2 out]
          }
          frame True {
            w394 = T15."Disabled" ("Disabled")
            n271 = property on="Auto Start Test" class="Bool (strict)"("Visible"=FALSE) -> ()  [unwired: 2 in, 2 out]
            n272 = property on="FRICVALZ 2" class="Bool (strict)"("DisabledEnum"=w394) -> ()  [unwired: 2 in, 2 out]
            n273 = property on="FRICVALZ 4" class="Bool (strict)"("DisabledEnum"=w394) -> ()  [unwired: 2 in, 2 out]
            n274 = property on="FRICVALZ 3" class="Bool (strict)"("DisabledEnum"=w394) -> ()  [unwired: 2 in, 2 out]
          }
        }
      }
      event "Auto": Value Change {
        n275 = event-data() -> ()  [unwired: 1 in, 6 out]
        n276 = stacked-sequence {
          frame #0 {
            n277 = local write "FILE"("") -> ()
          }
          frame #1 {
            n278 = Get Date/Time In Seconds() -> (seconds since 1Jan1904=w400:timestamp)
            n279 = Format Into String(format string="%<%I_%M_%S_%p_%d_%B_%Y>T", w400) -> (resulting string=w399:string)  [unwired: 2 in, 1 out]
            n280 = local write "FILE"(w399) -> ()
          }
        }
        n281 = local read "Auto"() -> (w397:bool)
        n282 = Not(x=w397) -> (.not. x?=w396:bool)
        n283 = local write "Auto"(w396) -> ()
      }
      event "Auto Start Test": Value Change {
        n284 = event-data() -> ()  [unwired: 1 in, 6 out]
        n285 = local read "Auto Start Test"() -> (w403:bool)
        n286 = case shown="True" w403 {
          frame False {
            w404 = T15."Enabled" ("Disabled")
            w408 = "" ("FILE")
            n287 = local write "Main Tab"(T2."Adv Scar" ("Main Tab")) -> ()
            n288 = local write "Main Dashboard Buttons"(T1."Imaging" ("Main Dashboard Buttons")) -> ()
            n289 = property on="RUN" class="Bool (strict)"("Visible"=TRUE) -> ()  [unwired: 2 in, 2 out]
            n290 = local write "TEST FILE NAM,E SAVED"(FALSE ("TEST FILE NAM,E SAVED")) -> ()
            n291 = local write "Fuel Discription :"(w408) -> ()
            n292 = local write "Batch Ref Num :"(w408) -> ()
            n293 = local write "Remarks :"(w408) -> ()
            n294 = local write "FILE"(w408) -> ()
            n295 = property on="FRICVALZ 2" class="Bool (strict)"("DisabledEnum"=w404) -> ()  [unwired: 2 in, 2 out]
            n296 = property on="FRICVALZ 4" class="Bool (strict)"("DisabledEnum"=w404) -> ()  [unwired: 2 in, 2 out]
            n297 = property on="FRICVALZ 3" class="Bool (strict)"("DisabledEnum"=w404) -> ()  [unwired: 2 in, 2 out]
          }
          frame True {
            w410 = T15."Disabled" ("Disabled")
            n298 = property on="RUN" class="Bool (strict)"("Visible"=FALSE) -> ()  [unwired: 2 in, 2 out]
            n299 = property on="FRICVALZ 2" class="Bool (strict)"("DisabledEnum"=w410) -> ()  [unwired: 2 in, 2 out]
            n300 = property on="FRICVALZ 4" class="Bool (strict)"("DisabledEnum"=w410) -> ()  [unwired: 2 in, 2 out]
            n301 = property on="FRICVALZ 3" class="Bool (strict)"("DisabledEnum"=w410) -> ()  [unwired: 2 in, 2 out]
          }
        }
      }
      event "FILE", "USERNAME", "USER ID": Mouse Enter {
        n302 = event-data() -> ()  [unwired: 1 in, 4 out]
        n303 = dll-call lib="kernel32.dll" fn="Wow64DisableWow64FsRedirection"("OldValue"=0) -> (error out=w417:errorcluster, "OldValue"=w415:i32)  [unwired: 4 in, 1 out]
        n304 = call <vilib>:"System Exec.vi"("run minimized? (F)"=TRUE, "error in (no error)"=w417, "command line"="C:\\Program Files\\Common Files\\Microsoft Shared\\Ink\\TabTip.exe") -> ("error out"=w416:errorcluster)  [unwired: 5 in, 3 out]
        n305 = dll-call lib="kernel32.dll" fn="Wow64EnableWow64FsRedirection"(error in=w416, "OldValue"=w415) -> ()  [unwired: 4 in, 2 out]
      }
      event "EDIT": Value Change {
        n306 = event-data() -> ()  [unwired: 1 in, 6 out]
        n307 = local read "EDIT"() -> (w418:bool)
        n308 = case shown="False" w418 {
          frame False {
            n309 = control-ref of="This VI"() -> (w435:refnum<vi>)
            n310 = property class="VI"(reference=w435) -> (reference out=w426:refnum<vi>, error out=w430:errorcluster, "Panel"=w434:refnum<vi>)  [unwired: 1 in]
            n311 = property class="Pnl"(reference=w434, error in=w430) -> (reference out=w428:refnum<vi>, error out=w431:errorcluster, "Panes[]"=w433:refnum<vi>[])
            n312 = for {
              tunnel: w433 -> [w441] mode=indexing
              tunnel: T17."Always Off" ("Horizontal Scrollbar Visibility") -> [w440]
              tunnel: w431 -> [w437]
              tunnel: [w436] -> w429
              n313 = property class="Pane"(reference=w441, error in=w437, "HorizScrollbarVisibility"=w440) -> (reference out=w438:refnum<vi>, error out=w439:errorcluster)
              n314 = Close Reference(reference=w438, error in (no error)=w439) -> (error out=w436:errorcluster)
            }
            n315 = Close Reference(reference=w428, error in (no error)=w429) -> (error out=w427:errorcluster)
            n316 = Close Reference(reference=w426, error in (no error)=w427) -> (error out=w421:errorcluster)
            "error out 7" <- w421
            n317 = call <vilib>:"Clear Errors.vi"("error in (no error)"=w421) -> ("error out"=w420:errorcluster)  [unwired: 5 in, 1 out]
            n318 = local write "Service Password enable"(FALSE ("Service Password enable")) -> ()
            n319 = call <userlib>:"Fit VI window to Largest Dec.vi"("error in (no error)"=w420, "border spacing (2 px)"=1) -> ("error out"=w425:errorcluster, "dup VI Ref"=w423:refnum<vi>)  [unwired: 4 in]
            n320 = invoke on="Invoke Node" class="VI" method="FP.Run-Time Position.Maximized"(reference=w423, error in=w425) -> (error out=w424:errorcluster)  [unwired: 2 in, 3 out]
            n321 = call <vilib>:"Clear Errors.vi"("error in (no error)"=w424) -> ()  [unwired: 5 in, 2 out]
          }
          frame True {
          }
        }
      }
      event "Headen Service Button": Value Change {
        n322 = event-data() -> ()  [unwired: 1 in, 6 out]
        n323 = local read "Headen Service Button"() -> (w442:bool)
        n324 = case shown="True" w442 {
          frame False {
            n325 = property on="Password 3" class="Clust (strict)"("Visible"=FALSE) -> ()  [unwired: 2 in, 2 out]
            n326 = property on="Service Password Log" class="Str"("Visible"=FALSE) -> ()  [unwired: 2 in, 2 out]
          }
          frame True {
            n327 = property on="Password 3" class="Clust (strict)"("Visible"=TRUE) -> ()  [unwired: 2 in, 2 out]
            n328 = property on="Service Password Log" class="Str"("Visible"=TRUE) -> ()  [unwired: 2 in, 2 out]
          }
        }
      }
      event "Password 3.Service Password": Value Change {
        n329 = event-data() -> ()  [unwired: 1 in, 6 out]
        n330 = Unbundle By Name("Password 3") -> ("Service Password"=w449:string)
        n331 = call <vilib>:"Trim Whitespace.vi"("string"=w449) -> ("trimmed string"=w447:string)  [unwired: 1 in]
        n332 = Equal?(x=w447, y="Service@123") -> (x = y?=w448:bool)
        n333 = case shown="False" w448 {
          selector: w448 -> [w452 w454]
          frame False {
            n334 = local write "Service Password enable"(w452) -> ()
            n335 = property on="Service Password Log" class="Str"("Visible"=TRUE) -> ()  [unwired: 2 in, 2 out]
          }
          frame True {
            n336 = property on="Service Password Log" class="Str"("Visible"=FALSE) -> ()  [unwired: 2 in, 2 out]
            "Service Password enable" <- w454
          }
        }
      }
      event "Sign In": Value Change {
        w456 = FALSE ("Visible")
        n337 = event-data() -> ()  [unwired: 1 in, 6 out]
        n338 = property on="About" class="Clust (strict)"("Visible"=w456) -> ()  [unwired: 2 in, 2 out]
        n339 = property on="Password 3" class="Clust (strict)"("Visible"=w456) -> ()  [unwired: 2 in, 2 out]
        n340 = property on="Service Password Log" class="Str"("Visible"=FALSE) -> ()  [unwired: 2 in, 2 out]
      }
      event "Info": Value Change {
        n341 = event-data() -> ()  [unwired: 1 in, 6 out]
        n342 = local read "Info"() -> (w458:bool)
        n343 = case shown="False" w458 {
          frame False {
            n344 = property on="About" class="Clust (strict)"("Visible"=FALSE) -> ()  [unwired: 2 in, 2 out]
          }
          frame True {
            n345 = property on="About" class="Clust (strict)"("Visible"=TRUE) -> ()  [unwired: 2 in, 2 out]
          }
        }
      }
      event "Quit": Value Change {
        n346 = event-data() -> ()  [unwired: 1 in, 6 out]
      }
    }
    n347 = Wait (ms)(milliseconds to wait=u32 100) -> ()  [unwired: 1 out]
  }
  n348 = local write "Auto stop temp"(w4) -> ()
  n349 = local write "main tab sub"(enum32{"Page 1", "Page 2"}."Page 1" ("main tab sub")) -> ()
  n350 = while {
    stop <- w488 stop-if-true
    w471 = errorcluster {"status"=FALSE, "code"=0, "source"=""} ("error in (no error) 3")
    # "this loop is for manual report generation"
    n351 = local read "Confirm Measrurement"() -> (w470:bool)
    n352 = case shown="True" w470 {
      selector: w470 -> [_ w578]
      tunnel: errorcluster {"status"=FALSE, "code"=0, "source"=""} ("error in (no error) 3") -> [_ w579]
      tunnel: [_ w577] -> _
      frame False {
      }
      frame True {
        n353 = stacked-sequence {
          tunnel: w579 -> [_ w610 _]
          tunnel: w578 -> [_ _ w709]
          tunnel: [_ w598 _] -> w577
          frame #0 {
            n354 = String To Path(string="C:\\LAB-IQ\\Image Calibrate v01.dcf") -> (path=w582:path)
            n355 = Open/Create/Replace File ("Open File")(file path (use dialog)=w582) -> (refnum out=w583:refnum<file>)  [unwired: 5 in, 2 out]
            n356 = for {
              N: 4 -> [_]
              tunnel: w583 -> [w589]
              i -> [w585]
              n357 = Read from Text File ("Read File")(file (use dialog)=w589) -> (text=w590:string)  [unwired: 3 in, 3 out]
              n358 = String Subset(string=w590, offset (0)=6, length (rest)=10 ("length (rest)")) -> (substring=w586:string)
              n359 = Fract/Exp String To Number(string=w586) -> (number=w584:dbl)  [unwired: 3 in, 1 out]
              n360 = case shown="3" w585 {
                tunnel: w584 -> [w591 w592 _ w593 _]
                frame 0 {
                  n361 = local write "5x Gain"(w591) -> ()
                }
                frame 1 {
                  n362 = local write "10x Gain"(w592) -> ()
                }
                frame 2 {
                }
                frame 3 {
                  n363 = local write "100x gain"(w593) -> ()
                }
                frame 4, Default {
                }
              }
            }
          }
          frame #1 {
            n364 = local read "Magnification :"() -> (w603:string)
            n365 = case shown="\"10x\"" w603 {
              tunnel: [w645 w646] -> w601
              frame "5x", Default {
                n366 = local read "5x Gain"() -> (w645:dbl)
              }
              frame "10x" {
                # "5x"
                n367 = local read "10x Gain"() -> (w646:dbl)
              }
            }
            n368 = call "IMAGE ANALYSIS.vi"("Enum"=POST_ANALYSIS_ENUM."GET MEASUREMENTS", "error in"=w610) -> ("error out"=w617:errorcluster)  [unwired: 8 in, 1 out]
            n369 = call "Stall Data Flow.vim"("value in"=w617, "milliseconds to wait"=u32 1000) -> ("value out"=w616:errorcluster)  [unwired: 1 out]
            n370 = local read "Test File List :"() -> (w614:string)
            n371 = call "IMAGE ANALYSIS.vi"("Enum"=POST_ANALYSIS_ENUM."READ", "error in"=w616) -> ("error out"=w613:errorcluster, "data out"=w604:string)  [unwired: 8 in]
            n372 = Match Pattern(string=w604, regular expression="\"type\": ") -> (after substring=w608:string)  [unwired: 1 in, 3 out]
            n373 = call "IMAGE PATH CREATION PY.vi"("error in (no error)"=w613, "File Name :"=w614) -> ("error out"=w612:errorcluster, "File Path"=w600:path, "File Path String:"=w595:string)  [unwired: 7 in]
            n374 = Match Pattern(string=w608, regular expression=",") -> (before substring=w594:string)  [unwired: 1 in, 3 out]
            n375 = local read "Calibration Tab"() -> (w597:enum32{"Measrument", "Calibrate"})
            n376 = call "Stall Data Flow.vim"("value in"=w612, "milliseconds to wait"=u32 250) -> ("value out"=w596:errorcluster)  [unwired: 1 out]
            n377 = Equal?(x=w594, y="\"rectangle\"") -> (x = y?=w605:bool)
            n378 = case shown="False" w605 {
              tunnel: w604 -> [w651 w706]
              tunnel: w601 -> [_ w697]
              tunnel: cluster{"major":dbl, "minor":dbl, "average":dbl} {"major"=0.0, "minor"=0.0, "average"=0.0} -> [w649 w693]
              tunnel: [w648 w690] -> w599
              tunnel: w594 -> [w650 _]
              tunnel: w601 -> [w647 _]
              frame False {
                n379 = Equal?(x=w650, y="\"line\"") -> (x = y?=w652:bool)
                n380 = case shown="True" w652 {
                  tunnel: w651 -> [_ w667]
                  tunnel: w649 -> [w654 w666]
                  tunnel: [w654 w664] -> w648
                  tunnel: w647 -> [_ w663]
                  frame False {
                  }
                  frame True {
                    w662 = 0.0 ("Major Axis")
                    n381 = Match Pattern(string=w667, regular expression="\"length_px\":") -> (after substring=w665:string)  [unwired: 1 in, 3 out]
                    n382 = property on="Major Axis" class="DigNum (strict)"("Caption.Text"="") -> ()  [unwired: 2 in, 2 out]
                    n383 = property on="Minor Axis" class="DigNum (strict)"("Caption.Text"="") -> ()  [unwired: 2 in, 2 out]
                    n384 = property on="Average" class="DigNum (strict)"("Caption.Text"="Line") -> ()  [unwired: 2 in, 2 out]
                    n385 = Fract/Exp String To Number(string=w665, default (0 dbl)=0.0 ("default (0 DBL)")) -> (number=w661:dbl)  [unwired: 2 in, 1 out]
                    "Pixel Value" <- w661
                    n386 = Multiply(x=w661, y=w663) -> (x*y=w674:dbl)
                    n387 = Multiply(x=w674, y=1000.0) -> (x*y=w657:dbl)
                    n388 = Divide(x=w657, y=1000.0) -> (x/y=w660:dbl)
                    n389 = local write "Measurment (mm)"(w660) -> ()
                    n390 = Bundle By Name(cluster=w666, "average"=w657) -> (w664:cluster{"major":dbl, "minor":dbl, "average":dbl})
                    n391 = Number To Fractional String(number=w657, precision (6)=i16 1) -> (F-format string=w656:string)  [unwired: 2 in]
                    n392 = local write "Minor Axis"(w662) -> ()
                    n393 = local write "Major Axis"(w662) -> ()
                    n394 = Fract/Exp String To Number(string=w656) -> (number=w655:dbl)  [unwired: 3 in, 1 out]
                    n395 = local write "Average"(w655) -> ()
                  }
                }
              }
              frame True {
                w694 = 1000.0 ("y")
                w700 = 0.0 ("default (0 DBL)")
                n396 = Match Pattern(string=w706, regular expression=" \"width_px\":") -> (after substring=w704:string)  [unwired: 1 in, 3 out]
                n397 = Match Pattern(string=w704, regular expression="\"height_px\":") -> (before substring=w702:string, after substring=w701:string)  [unwired: 1 in, 2 out]
                n398 = Fract/Exp String To Number(string=w702, default (0 dbl)=w700) -> (number=w699:dbl)  [unwired: 2 in, 1 out]
                n399 = Fract/Exp String To Number(string=w701, default (0 dbl)=w700) -> (number=w698:dbl)  [unwired: 2 in, 1 out]
                n400 = Multiply(x=w699, y=w697) -> (x*y=w696:dbl)
                n401 = Multiply(x=w698, y=w697) -> (x*y=w695:dbl)
                n402 = Multiply(x=w696, y=w694) -> (x*y=w680:dbl)
                n403 = Multiply(x=w695, y=w694) -> (x*y=w678:dbl)
                n404 = Add(x=w680, y=w678) -> (x+y=w692:dbl)
                n405 = property on="Major Axis" class="DigNum (strict)"("Caption.Text"="Major Axis") -> ()  [unwired: 2 in, 2 out]
                n406 = property on="Minor Axis" class="DigNum (strict)"("Caption.Text"="Minor Axis") -> ()  [unwired: 2 in, 2 out]
                n407 = property on="Average" class="DigNum (strict)"("Caption.Text"="Average") -> ()  [unwired: 2 in, 2 out]
                n408 = Divide(x=w692, y=2.0) -> (x/y=w676:dbl)
                n409 = Bundle By Name(cluster=w693, "major"=w680, "minor"=w678, "average"=w676) -> (w690:cluster{"major":dbl, "minor":dbl, "average":dbl})
                n410 = Number To Fractional String(number=w678, precision (6)=i16 1) -> (F-format string=w685:string)  [unwired: 2 in]
                n411 = Number To Fractional String(number=w676, precision (6)=i16 1) -> (F-format string=w686:string)  [unwired: 2 in]
                n412 = Number To Fractional String(number=w680, precision (6)=i16 1) -> (F-format string=w684:string)  [unwired: 2 in]
                n413 = Fract/Exp String To Number(string=w685) -> (number=w677:dbl)  [unwired: 3 in, 1 out]
                n414 = Fract/Exp String To Number(string=w686) -> (number=w675:dbl)  [unwired: 3 in, 1 out]
                n415 = Fract/Exp String To Number(string=w684) -> (number=w679:dbl)  [unwired: 3 in, 1 out]
                n416 = local write "Major Axis"(w679) -> ()
                n417 = local write "Average"(w675) -> ()
                n418 = local write "Minor Axis"(w677) -> ()
              }
            }
            n419 = case shown="\"Measrument\", Default" w597 {
              tunnel: w600 -> [w624 _]
              tunnel: w599 -> [w623 _]
              tunnel: [w620 w644] -> w598
              tunnel: w596 -> [w622 w644]
              tunnel: w595 -> [w621 _]
              frame "Measrument", Default {
                n420 = stacked-sequence {
                  tunnel: w624 -> [w637 _]
                  tunnel: w623 -> [w635 _]
                  tunnel: w622 -> [w633 _]
                  tunnel: w621 -> [w632 _]
                  tunnel: [w627 _] -> w620
                  frame #0 {
                    n421 = call "IMAGE ANALYSIS.vi"("Enum"=POST_ANALYSIS_ENUM."SAVE IMAGE", "error in"=w633, "IMAGE FILE PATH"=w632) -> ("error out"=w631:errorcluster)  [unwired: 7 in, 1 out]
                    n422 = local read "Test File List :"() -> (w639:string)
                    n423 = call "IMAGE ANALYSIS.vi"("Enum"=POST_ANALYSIS_ENUM."MINIMIZE UI", "error in"=w631) -> ("error out"=w629:errorcluster)  [unwired: 8 in, 1 out]
                    n424 = Bundle By Name(cluster=T20 {"File Name"="", "Test Method"="", "Operator"="", "Fuel Description"="", "Date and time"=""} ("Main Ref"), "File Name"=w639) -> (w640:T20)
                    n425 = call "duf file read.vi"("error in (no error)"=w629, "Main Ref"=w640) -> ("error out"=w638:errorcluster, "Main Ref 2"=w636:T20)  [unwired: 8 in]
                    n426 = call "DETECTION REPORT for manual.vi"("error in (no error)"=w638, "return value 3"=w635, "Image File Path"=w637, "Main Ref"=w636) -> ("error out"=w634:errorcluster)  [unwired: 7 in]
                    n427 = call <vilib>:"Clear Errors.vi"("error in (no error)"=w634) -> ("error out"=w625:errorcluster)  [unwired: 5 in, 1 out]
                    n428 = call "IMAGE ANALYSIS.vi"("Enum"=POST_ANALYSIS_ENUM."MINIMIZE UI", "error in"=w625) -> ("error out"=w627:errorcluster)  [unwired: 8 in, 1 out]
                  }
                  frame #1 {
                    n429 = local write "Main Tab"(T2."HOME" ("Main Tab")) -> ()
